vi "Mandelbrot_CuLab.vi"() -> ()   [LabVIEW 2020]
uses:
  <vilib>/Ngene/CuLab - GPU Accelerated Toolkit/Toolkit/Low_Level/GPU_Wrapper/culab_comparison/Controls/culab_bool_op_2in.ctl
  <vilib>/Ngene/CuLab - GPU Accelerated Toolkit/Toolkit/Low_Level/GPU_Wrapper/culab_comparison/Controls/culab_bool_neg_inputs.ctl
  <vilib>/Ngene/CuLab - GPU Accelerated Toolkit/Toolkit/Low_Level/GPU_Wrapper/culab_comparison/Controls/culab_comp_mode_2in.ctl
  acdee1ab-0b82-4047-983d-88c3d57dfc2c.vi
  <vilib>/Analysis/1siggen.llb/Ramp Pattern by Samples.vi
  <vilib>/Ngene/CuLab - GPU Accelerated Toolkit/Toolkit/Low_Level/Tensor_Classes/T_Children/T2D/T2D_Children/T2D_I16/Pull.vi
  5424d61b-997c-4bc6-ad91-23142d452257.vi
  <vilib>/Ngene/CuLab - GPU Accelerated Toolkit/Toolkit/Low_Level/GPU_Wrapper/cudart/Memory/PULL/2D/cudart_PULL_Data(I16_2D).vi
  <vilib>/Ngene/CuLab - GPU Accelerated Toolkit/Toolkit/Low_Level/Tensor_Classes/T_Children/T2D/T2D_Children/T2D_DBL/T2D_DBL.lvclass
  C:/Program Files/National Instruments/LabVIEW 2020/vi.lib/Ngene/CuLab - GPU Accelerated Toolkit/Toolkit/Low_Level/Tensor_Classes/T_Children/T2D/T2D.lvclass
  <vilib>/Ngene/CuLab - GPU Accelerated Toolkit/Toolkit/Low_Level/Tensor_Classes/T_Children/T2D/T2D_Children/T2D_U8/T2D_U8.lvclass
  <vilib>/Ngene/CuLab - GPU Accelerated Toolkit/Toolkit/Low_Level/Tensor_Classes/T_Children/T2D/T2D_Children/T2D_I16/T2D_I16.lvclass
  C:/Program Files/National Instruments/LabVIEW 2020/vi.lib/Ngene/CuLab - GPU Accelerated Toolkit/Toolkit/Low_Level/Tensor_Classes/Tensor.lvclass
  <vilib>/Ngene/CuLab - GPU Accelerated Toolkit/Toolkit/Low_Level/Tensor_Classes/T_Children/T2D/T2D_Children/T2D_U8/Create.vi
  <vilib>/Ngene/CuLab - GPU Accelerated Toolkit/Toolkit/Low_Level/Tensor_Classes/T_Children/T2D/T2D_Children/T2D_I16/Create.vi
  <vilib>/Ngene/CuLab - GPU Accelerated Toolkit/Toolkit/API/Array/Initialize Array/T2D/CU_Initialize Array_T2D_DBL.vi
  <vilib>/Ngene/CuLab - GPU Accelerated Toolkit/Toolkit/API/Array/Array Size/CU_Array_Size_T2D.vi
  <vilib>/Ngene/CuLab - GPU Accelerated Toolkit/Toolkit/API/Signal Processing/Signal Generation/Ramp Pattern/T1D/CU_Ramp_Pattern_T1D_DBL.vi
  <vilib>/Ngene/CuLab - GPU Accelerated Toolkit/Toolkit/API/Numeric/Add Broadcast/CU_Add_Broadcast_DBL.vi
  <vilib>/Ngene/CuLab - GPU Accelerated Toolkit/Toolkit/API/Numeric/Complex  (API)/Re Im To Complex/T2D/CU_Re_Im_To_Complex_T2D_DBL.vi
  <vilib>/Ngene/CuLab - GPU Accelerated Toolkit/Toolkit/API/Numeric/Multiply/T2D/CU_MultiplyC_T2D_CDB.vi
  <vilib>/Ngene/CuLab - GPU Accelerated Toolkit/Toolkit/API/Numeric/Multiply/T2D/CU_MultiplyC_T2D_U8.vi
  <vilib>/Ngene/CuLab - GPU Accelerated Toolkit/Toolkit/API/Numeric/Multiply/T2D/CU_MultiplyC_T2D_I16.vi
  <vilib>/Ngene/CuLab - GPU Accelerated Toolkit/Toolkit/API/Numeric/Square/T2D/CU_Square_T2D_CDB.vi
  <vilib>/Ngene/CuLab - GPU Accelerated Toolkit/Toolkit/API/Numeric/Add/T2D/CU_Add_T2D_CDB.vi
  <vilib>/Ngene/CuLab - GPU Accelerated Toolkit/Toolkit/API/Comparison/Compare_2_Inputs/T2D/CU_Compare_2InC_T2D_CDB.vi
  <vilib>/Ngene/CuLab - GPU Accelerated Toolkit/Toolkit/API/Boolean/Boolean_2in/T2D/CU_Boolean_2In_T2D_U8.vi
  <vilib>/Ngene/CuLab - GPU Accelerated Toolkit/Toolkit/API/Numeric/Conversion  (API)/I16/CU_To_I16_T2D.vi
  <vilib>/Ngene/CuLab - GPU Accelerated Toolkit/Toolkit/API/Numeric/Add/T2D/CU_Add_T2D_I16.vi
  <vilib>/Ngene/CuLab - GPU Accelerated Toolkit/Toolkit/Low_Level/Checkers/Check_Tensor_Ref.vi
  <vilib>/Ngene/CuLab - GPU Accelerated Toolkit/Toolkit/Low_Level/Tensor_Classes/Property/Get_Mem_Desc.vi
  <vilib>/Ngene/CuLab - GPU Accelerated Toolkit/Toolkit/Low_Level/Tensor_Classes/T_Children/T2D/Property/Get_Dims.vi
  <vilib>/Ngene/CuLab - GPU Accelerated Toolkit/Toolkit/Low_Level/GPU_Wrapper/cudart/Memory/Utils/cudart_get_type_size(inBytes).vi
  <vilib>/Ngene/CuLab - GPU Accelerated Toolkit/Toolkit/Low_Level/GPU_Wrapper/cudart/cudart_get_Error_String.vi
  <vilib>/Ngene/CuLab - GPU Accelerated Toolkit/Toolkit/CuLab.lvlib
  <vilib>/Analysis/NI_AALBase.lvlib
  C:/Program Files/National Instruments/LabVIEW 2020/vi.lib/Ngene/CuLab - GPU Accelerated Toolkit/Toolkit/Low_Level/Tensor_Classes/T_Children/T2D/T2D_Children/T2D_DBL/T2D_DBL.lvclass
  C:/Program Files/National Instruments/LabVIEW 2020/vi.lib/Ngene/CuLab - GPU Accelerated Toolkit/Toolkit/Low_Level/Tensor_Classes/T_Children/T2D/T2D_Children/T2D_U8/T2D_U8.lvclass
panel:
  out "Device":string="NVIDIA GeForce RTX 2080 Ti"
  out "Current Frame":i32=223
  out "Time Elapsed":dbl=23.5 format="%#_3fs"
  out "Total Frames":i32=224
  out "Current Iters":i32=1500
  in  "Zoom Stop":dbl=1e-05 format="%#.9g"
  in  "Zoom Start":dbl=0.95 format="%#.9g"
  in  "Iters. Stop":i32=1500
  out "Time per Frame":dbl=0.165 format="%#_3ps"
  out "Current Zoom":dbl=1e-05
  in  "y":dbl=0.13182590420533 format="%#_17g"
  in  "x":dbl=-0.743643887037151 format="%#_18g"
  out "Mandelbrot Graph":i16[][](graph)
  in  "Iters. Start":i32=500
  in  "Resolution":i32=500
  # "Mandelbrot CuLab"
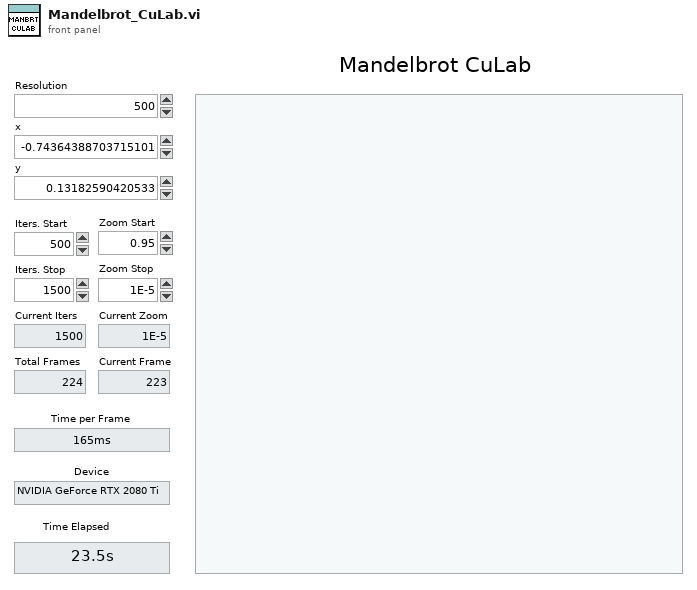
[diagram p1: front panel]
types:
  T1 = typedef "CuLab.lvlib/Properties.ctl" = cluster{"Device ID":i32, "Name":string}
  T2 = typedef "CuLab.lvlib/culab_comp_mode_2in.ctl" = enum8{"Equal?", "Not Equal?", "Greater?", "Greater Or Equal?", "Less?", "Less Or Equal?"}
  T3 = typedef "CuLab.lvlib/culab_bool_neg_inputs.ctl" = enum32{"None", "First Input", "Second Input", "Both"}
  T4 = typedef "CuLab.lvlib/culab_bool_op_2in.ctl" = enum32{"AND", "OR", "XOR", "NAND", "NOR", "XNOR", "Select X", "Select Y"}
  T5 = typedef "CuLab.lvlib/T2D_Dims.ctl" = cluster{"H":i32, "W":i32}
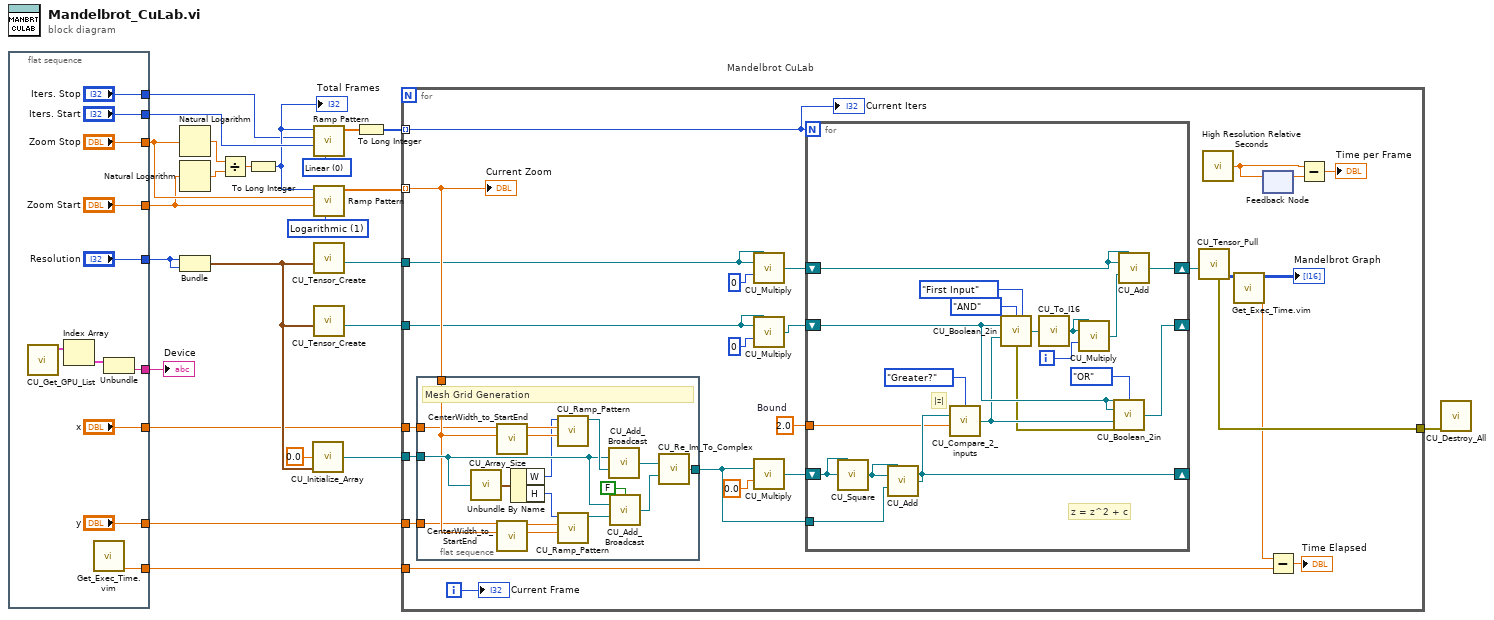
[diagram p0: block diagram]
diagram:
  w8 = u16 0 items=["Linear", "Logarithmic"] ("type")
  w7 = u16 1 items=["Linear", "Logarithmic"] ("type")
  # "Mandelbrot CuLab"
  n1 = flat-sequence {
    tunnel: ["Resolution"] -> w18
    tunnel: ["Iters. Start"] -> w13
    tunnel: ["Zoom Stop"] -> w10
    tunnel: ["Zoom Start"] -> w9
    tunnel: ["Iters. Stop"] -> w6
    tunnel: ["x"] -> w4
    tunnel: ["y"] -> w3
    tunnel: [w28] -> w2
    tunnel: [w25] -> w1
    frame #0 {
      n2 = call <vilib>:"CU_Get_GPU_List.vi"() -> ("Devices"=w27:T1[])  [unwired: 10 in, 1 out]
      n3 = Index Array(array=w27) -> (element=w26:T1)  [unwired: 1 in]
      n4 = call "Get_Exec_Time.vim"() -> ("T(n)"=w28:dbl)  [unwired: 7 in, 2 out]
      n5 = Unbundle(w26) -> ("Name"=w25:string)  [unwired: 1 out]
    }
  }
  n6 = Natural Logarithm(1:w10) -> (0:w15:dbl)
  n7 = Natural Logarithm(1:w9) -> (0:w16:dbl)
  n8 = Bundle("Resolution"=w18, "Resolution"=w18) -> (w5:cluster{"Resolution":i32, "Resolution":i32})  [unwired: 1 in]
  n9 = Divide(x=w15, y=w16) -> (x/y=w14:dbl)
  n10 = To Long Integer(number=w14) -> (32bit integer=w11:i32)
  "Total Frames" <- w11
  n11 = call-poly <vilib>:"CU_Initialize_Array.vi"("element"=0.0, "dimension sizes"=w5) -> ("initialized Tensor"=w22:refnum<class "T2D_DBL.lvclass">)  [unwired: 12 in, 1 out]
  n12 = call-poly <vilib>:"Ramp Pattern.vi"("type"=w8, "start"=w13, "end"=w6, "samples"=w11) -> ("Ramp Pattern"=w12:dbl[])  [unwired: 6 in, 1 out]
  n13 = call-poly <vilib>:"Ramp Pattern.vi"("type"=w7, "start"=w9, "end"=w10, "samples"=w11) -> ("Ramp Pattern"=w20:dbl[])  [unwired: 6 in, 1 out]
  n14 = call-poly <vilib>:"CU_Tensor_Create.vi"("T2D_Dims"=w5) -> ("T2D_I16 out"=w24:refnum<class "T2D_I16.lvclass">)  [unwired: 9 in, 1 out]
  n15 = call-poly <vilib>:"CU_Tensor_Create.vi"("T2D_Dims"=w5) -> ("T2D_U8 out"=w23:refnum<class "T2D_U8.lvclass">)  [unwired: 9 in, 1 out]
  n16 = To Long Integer(number=w12) -> (32bit integer=w21:i32[])
  n17 = for {
    tunnel: [w46] -> w19
    tunnel: w24 -> [w53]
    tunnel: w23 -> [w51]
    tunnel: w22 -> [w59]
    tunnel: w21 -> [w56] mode=indexing
    tunnel: w20 -> [w55] mode=indexing
    tunnel: w2 -> [w41]
    tunnel: w4 -> [w37]
    tunnel: w3 -> [w36]
    i -> [w39]
    w45 = sgl 2.0  # Bound
    n18 = flat-sequence {
      tunnel: [w69] -> w61
      tunnel: w59 -> [w68]
      tunnel: w55 -> [w65]
      tunnel: w37 -> [w64]
      tunnel: w36 -> [w63]
      frame #0 {
        # "Mesh Grid Generation"
        n19 = call-poly <vilib>:"CU_Array_Size.vi"("Tensor"=w68) -> ("T2D_Dims"=w67:T5)  [unwired: 14 in]
        n20 = call "CenterWidth_to_StartEnd.vi"("width"=w65, "Center"=w64) -> ("Start"=w77:dbl, "End"=w78:dbl)  [unwired: 8 in]
        n21 = call "CenterWidth_to_StartEnd.vi"("width"=w65, "Center"=w63) -> ("Start"=w75:dbl, "End"=w76:dbl)  [unwired: 8 in]
        n22 = Unbundle By Name(w67) -> ("W"=w62:i32, "H"=w66:i32)
        n23 = call-poly <vilib>:"CU_Ramp_Pattern.vi"("start"=w77, "end"=w78, "samples"=w62) -> ("Ramp Pattern"=w74:refnum<class "T1D_DBL.lvclass">)  [unwired: 7 in, 1 out]
        n24 = call-poly <vilib>:"CU_Ramp_Pattern.vi"("start"=w75, "end"=w76, "samples"=w66) -> ("Ramp Pattern"=w73:refnum<class "T1D_DBL.lvclass">)  [unwired: 7 in, 1 out]
        n25 = call-poly <vilib>:"CU_Add_Broadcast.vi"("x"=w68, "y"=w74) -> ("Dest out"=w71:refnum<class "T2D_DBL.lvclass">)  [unwired: 12 in, 1 out]
        n26 = call-poly <vilib>:"CU_Add_Broadcast.vi"("By Rows?"=FALSE, "x"=w68, "y"=w73) -> ("Dest out"=w72:refnum<class "T2D_DBL.lvclass">)  [unwired: 11 in, 1 out]
        n27 = call-poly <vilib>:"CU_Re_Im_To_Complex.vi"("x"=w71, "y"=w72) -> ("Dest out"=w69:refnum<class "T2D_CDB.lvclass">)  [unwired: 12 in, 1 out]
      }
    }
    n28 = call-poly <vilib>:"CU_Multiply.vi"("Dest in"=w53, "x"=w53, "y"=i16 0 ("Value")) -> ("Dest out"=w60:refnum<class "T2D_I16.lvclass">)  [unwired: 11 in, 1 out]
    n29 = call-poly <vilib>:"CU_Multiply.vi"("Dest in"=w51, "x"=w51, "y"=u8 0 ("element")) -> ("Dest out"=w52:refnum<class "T2D_U8.lvclass">)  [unwired: 11 in, 1 out]
    n30 = call-poly <vilib>:"CU_Multiply.vi"("x"=w61, "y"=sgl 0.0 ("start")) -> ("Dest out"=w49:refnum<class "T2D_CDB.lvclass">)  [unwired: 12 in, 1 out]
    n31 = for {
      N: w56 -> [_]
      shift-right: [w90] -> _
      shift-left: w49 -> [w93]
      tunnel: w61 -> [w95]
      shift-right: [w97] -> w47
      shift-left: w60 -> [w94]
      shift-right: [w96] -> _
      shift-left: w52 -> [w91]
      tunnel: w45 -> [w79]
      i -> [w80]
      # "|z|"
      # "z = z^2 + c"
      n32 = call-poly <vilib>:"CU_Square.vi"("Dest in"=w93, "x"=w93) -> ("Dest out"=w92:refnum<class "T2D_CDB.lvclass">)  [unwired: 12 in, 1 out]
      n33 = call-poly <vilib>:"CU_Add.vi"("Dest in"=w92, "x"=w92, "y"=w95) -> ("Dest out"=w90:refnum<class "T2D_CDB.lvclass">)  [unwired: 11 in, 1 out]
      n34 = call-poly <vilib>:"CU_Compare_2_inputs.vi"("Comp Mode"=culab_comp_mode_2in."Greater?", "x"=w90, "y"=w79) -> ("Dest out"=w86:refnum<class "T2D_U8.lvclass">)  [unwired: 11 in, 1 out]
      n35 = call-poly <vilib>:"CU_Boolean_2in.vi"("Bool Operation"=culab_bool_op_2in."AND", "Negate input/s?"=culab_bool_neg_inputs."First Input", "x"=w91, "y"=w86) -> ("Dest out"=w85:refnum<class "T2D_U8.lvclass">, "error out"=w82:errorcluster)  [unwired: 10 in]
      n36 = call-poly <vilib>:"CU_To_I16.vi"("Tensor in"=w85) -> ("Dest out"=w83:refnum<class "T2D_I16.lvclass">)  [unwired: 13 in, 1 out]
      n37 = call-poly <vilib>:"CU_Multiply.vi"("Dest in"=w83, "x"=w83, "y"=w80) -> ("Dest out"=w84:refnum<class "T2D_I16.lvclass">)  [unwired: 11 in, 1 out]
      n38 = call-poly <vilib>:"CU_Boolean_2in.vi"("Dest In"=w91, "Bool Operation"=culab_bool_op_2in."OR", "x"=w91, "y"=w86, "error in (no error)"=w82) -> ("Dest out"=w96:refnum<class "T2D_U8.lvclass">)  [unwired: 9 in, 1 out]
      n39 = call-poly <vilib>:"CU_Add.vi"("Dest in"=w94, "x"=w94, "y"=w84) -> ("Dest out"=w97:refnum<class "T2D_I16.lvclass">)  [unwired: 11 in, 1 out]
    }
    n40 = call-poly <vilib>:"CU_Tensor_Pull.vi"("T2D_I16 in"=w47) -> ("Dest out"=w43:i16[][], "error out"=w46:errorcluster)  [unwired: 8 in, 1 out]
    n41 = call <vilib>:"High Resolution Relative Seconds.vi"() -> ("relative seconds"=w44:dbl)
    n42 = call "Get_Exec_Time.vim"("error in (no error)"=w43) -> ("T(n)"=w42:dbl, "error out"=→"Mandelbrot Graph":i16[][])  [unwired: 6 in, 1 out]
    n43 = feedback #1() -> (w58:dbl)  [unwired: 1 in]
    n44 = feedback-in #1(w44) -> ()
    n45 = Subtract(x=w42, y=w41) -> (x-y=→"Time Elapsed":dbl)
    n46 = Subtract(x=w44, y=w58) -> (x-y=→"Time per Frame":dbl)
    "Current Zoom" <- w55
    "Current Iters" <- w56
    "Current Frame" <- w39
  }
  n47 = call <vilib>:"CU_Destroy_All.vi"("error in"=w19) -> ()  [unwired: 10 in, 1 out]
  "Device" <- w1
